vi "Interpolation Algo V1.vi"() -> (1 "SubRange":u16, 9 "MaxIndex":u16)   [LabVIEW 2013]
uses:
  Controls/Algorithm State.ctl
  <vilib>/Platform/TimedLoop/XDataNode/timing_clust.ctl
  <vilib>/Platform/TimedLoop/XDataNode/nitl_modes.ctl
  <vilib>/Platform/TimedLoop/XDataNode/wakeup.ctl
  <vilib>/rvi/Emulation/niFpgaSctlEmulationGetInTimedLoop.vi
  <vilib>/rvi/Emulation/niFpgaEmulationReportErrorSimple.vi
  <vilib>/rvi/Emulation/niFpgaGetClockAttributes.vi
  <vilib>/rvi/Emulation/niFpgaCriticalErrorInLSC.vi
  <vilib>/rvi/FIFO/Fifo_Resource/nirvififoEmulationReadFpgaImpl.vi
  <vilib>/rvi/DataTransferAndStorage/Container/Common/niFpgaContainerGetUniqueNameForEmu.vi
  <vilib>/rvi/interface/RandomDataEmulation/nirviRandomDataFPGAFIFO.vi
  <vilib>/rvi/interface/RandomDataEmulation/niFpgaRandomDataHandleErrors.vi
  <vilib>/rvi/Emulation/niFpgaProcessEmulError.vi
  LIDAR V2 Globals.vi
  <vilib>/rvi/FIFO/Fifo_Resource/nirvififoEmulationWriteFpgaImpl.vi
  <vilib>/rvi/Memory/Memory_Emulation/nirvimemoryFastEmulationFpgaImpl.vi
  <instcachedir>/0/nirvimemoryFastEmulationFpgaImpl_5FBAB50466BC4C939F684F8805638BFC.lvgen/nirvimemoryFastEmulationFpgaImpl_5FBAB50466BC4C939F684F8805638BFC_005.vi
  <vilib>/rvi/Memory/Memory_Emulation/nirvimemoryFastEmulation.vi
  <vilib>/rvi/Memory/Memory_Emulation/nirvimemoryEmulation.vi
  <instcachedir>/0/nirvimemoryFastEmulationFpgaImpl_5FBAB50466BC4C939F684F8805638BFC.lvgen/nirvimemoryFastEmulationFpgaImpl_5FBAB50466BC4C939F684F8805638BFC_007.vi
  <vilib>/Platform/TimedLoop/XDataNode/XDataNode.xnode
  <vilib>/rvi/DataTransferAndStorage/Container/XNode/niFpgaContainer.xnode
  <vilib>/rvi/FIFO/Fifo_Resource/nirvififoEmulationRead.vi
  <vilib>/rvi/interface/RandomDataEmulation/nirviRandomDataFpgaReadWriteTemplate.vi
  <vilib>/rvi/FIFO/Fifo_Resource/nirvififoEmulationWrite.vi
  <vilib>/rvi/FXPMathLib/FxpMul/XNode/nifxpmath_Multiplier.xnode
  <vilib>/rvi/FXPMathLib/FxpAdd/XNode/nifxpmath_Add.xnode
  <vilib>/Platform/TimedLoop/XDataNode/XDNodeRunTimeDep.lvlib
  <vilib>/rvi/FXPMathLib/sim/FxpSim.dll
panel:
  out "LedInfo":u16
  out "SumMaxValue":fxp<+/-,22,22>
  out "Buffer":fxp<+/-,22,22>[](array[numeric])
  out "AlgoState":T1
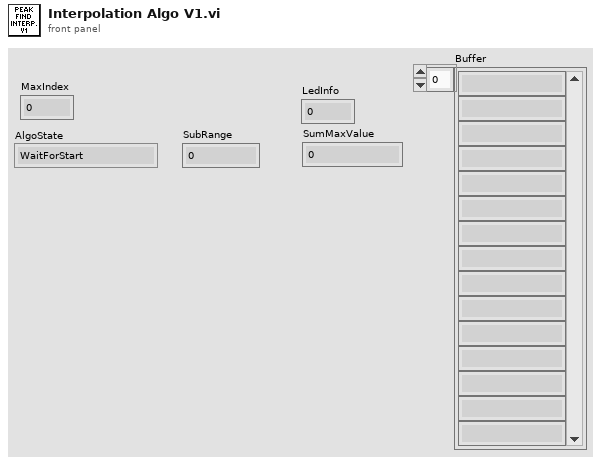
[diagram p1: front panel]
types:
  T1 = typedef "Algorithm State.ctl" = enum16{"WaitForStart", "GetNextSignalElement", "WaitForNextSignalElem", "MultWithSinc", "CalcMax"}
  T2 = typedef "XDNodeRunTimeDep.lvlib/timing_clust.ctl" = cluster{"Expected End [f-1]":u64, "Actual End [f-1]":u64, "Finished Late? [f-1]":bool, "Expected End [i-1]":u64, "Actual End [i-1]":u64, "Finished Late? [i-1]":bool, "Expected Start [i]":u64, "Actual Start [i]":u64, "Expected Start [f]":u64, "Actual Start [f]":u64, "Source Name":string, "Structure Name":string, "Period":i64, "Deadline":i64, "Offset":i64, "Start":i64, "Priority":i32, "Timeout":i32, "Mode":T3, "Wakeup Reason":T4, "Error":errorcluster, "Source Type":string, "Secondary Source Type":string, "Global End Time":u64, "Global Start Time":u64, "Frame Duration":u64, "Iteration Duration":u64, "Assigned CPU":i32, "I/O Scan Engine Mode":u32}
  T3 = typedef "XDNodeRunTimeDep.lvlib/nitl_modes.ctl" = enum32{"No Change", "Process missed periods, maintain original phase", "Discard missed periods, maintain original phase", "Process missed periods, ignore original phase", "Discard missed periods, ignore original phase"}
  T4 = typedef "XDNodeRunTimeDep.lvlib/wakeup.ctl" = enum32{"Normal", "Aborted", "Asynchronous wakeup", "Timing source error", "Timed loop error", "Timeout"}
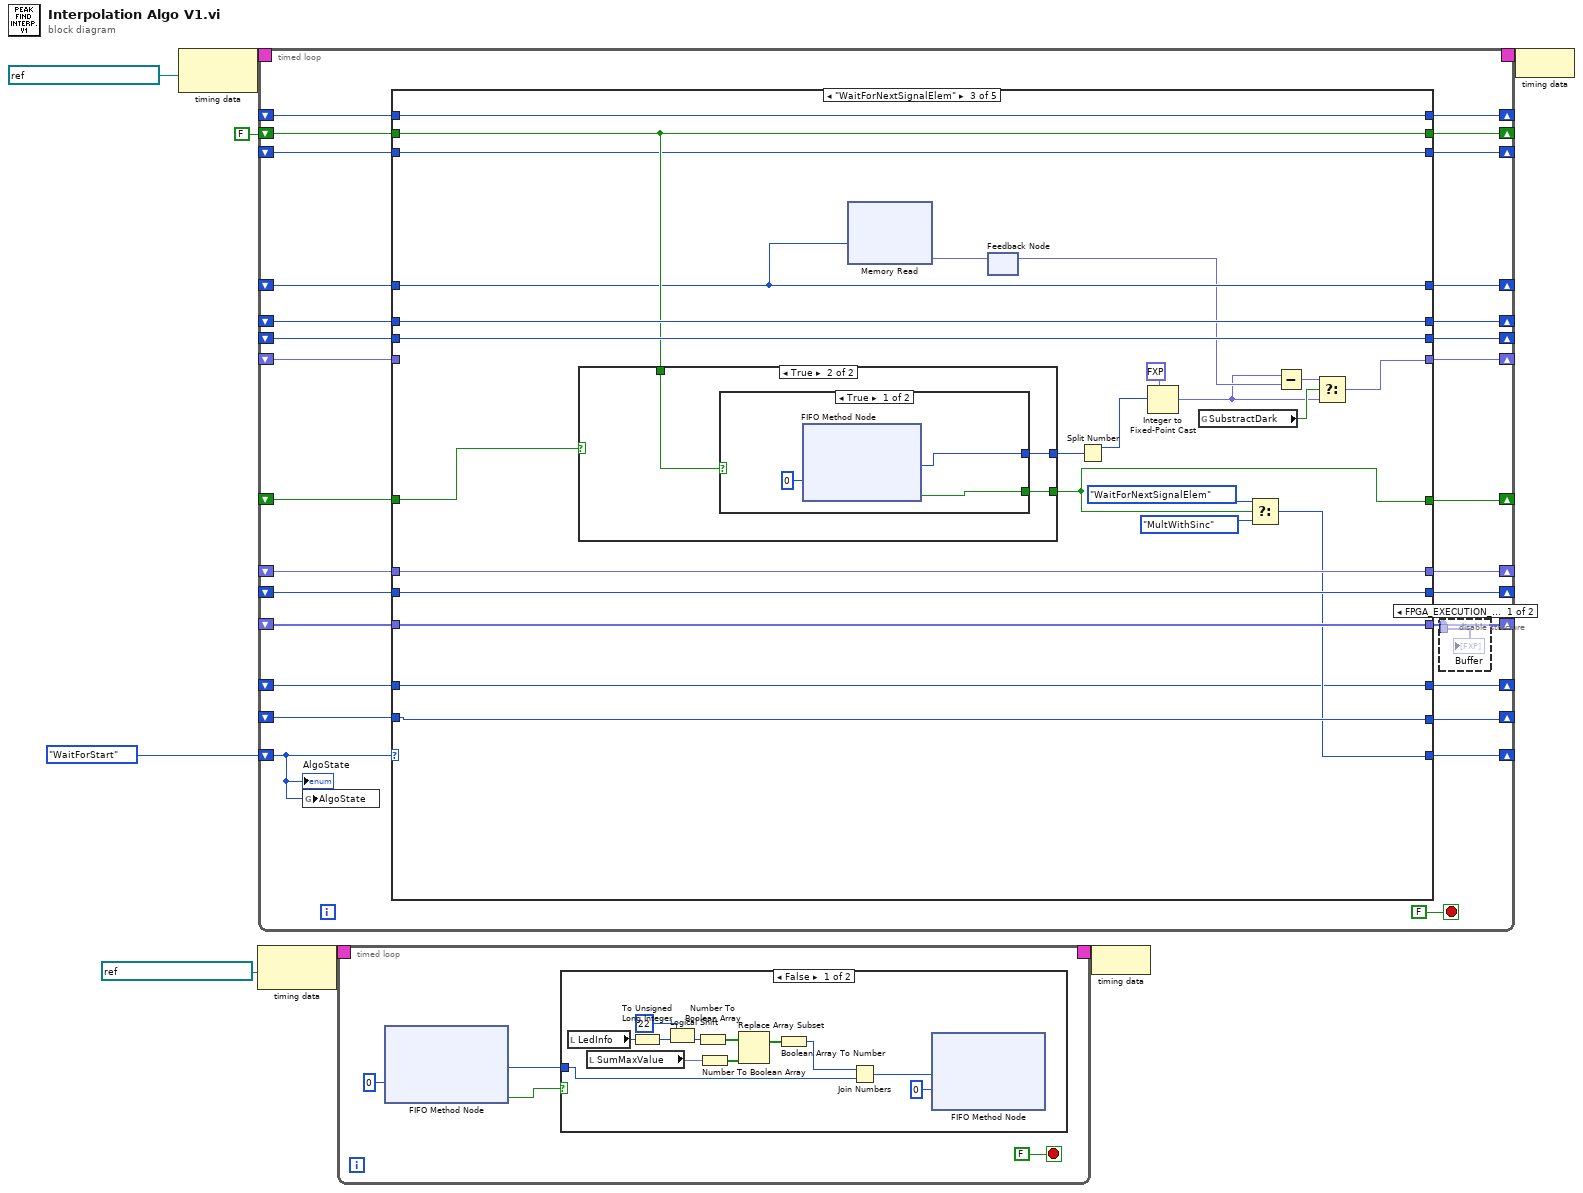
[diagram p0: block diagram]
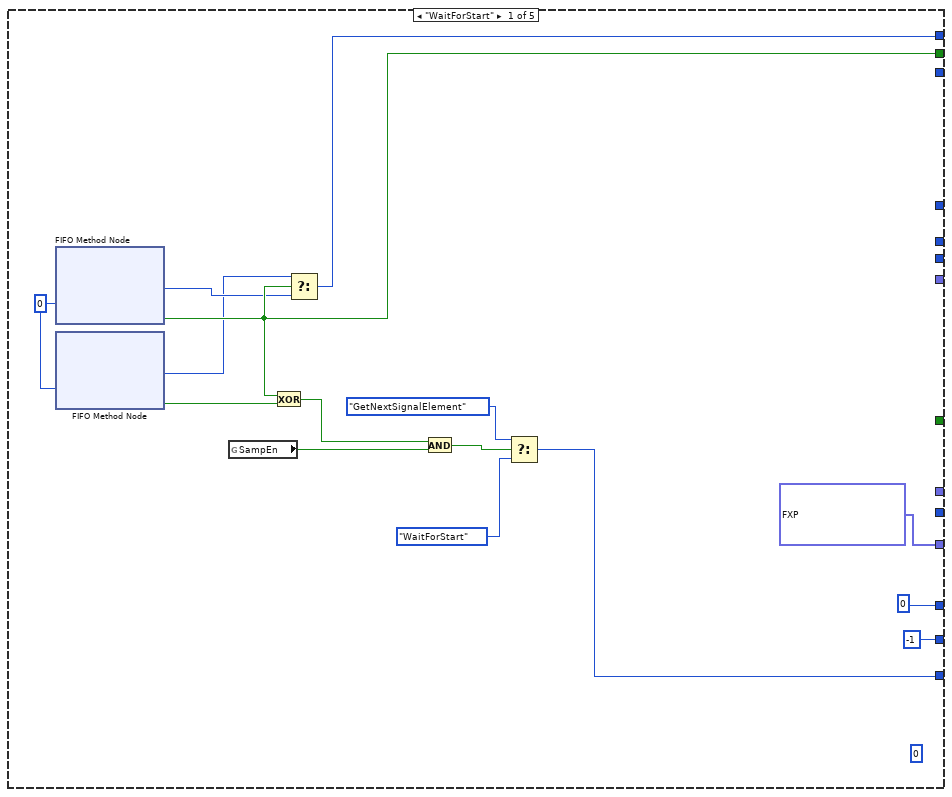
[diagram p4: hidden frame]
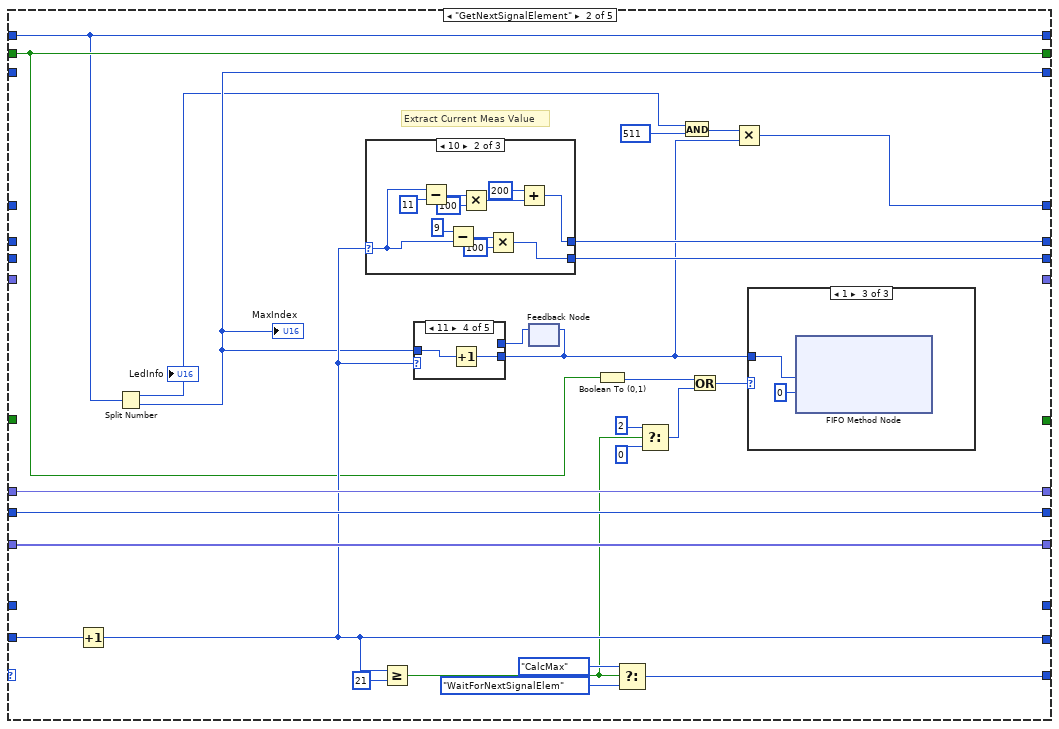
[diagram p5: hidden frame]
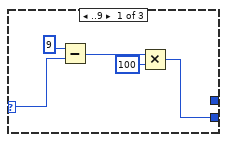
[diagram p6: hidden frame]
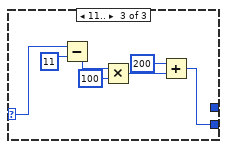
[diagram p7: hidden frame]
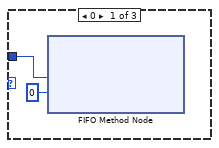
[diagram p8: hidden frame]
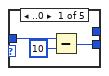
[diagram p10: hidden frame]
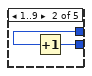
[diagram p11: hidden frame]
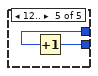
[diagram p13: hidden frame]
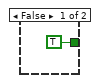
[diagram p14: hidden frame]
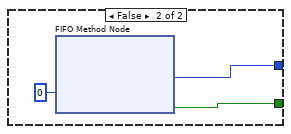
[diagram p15: hidden frame]
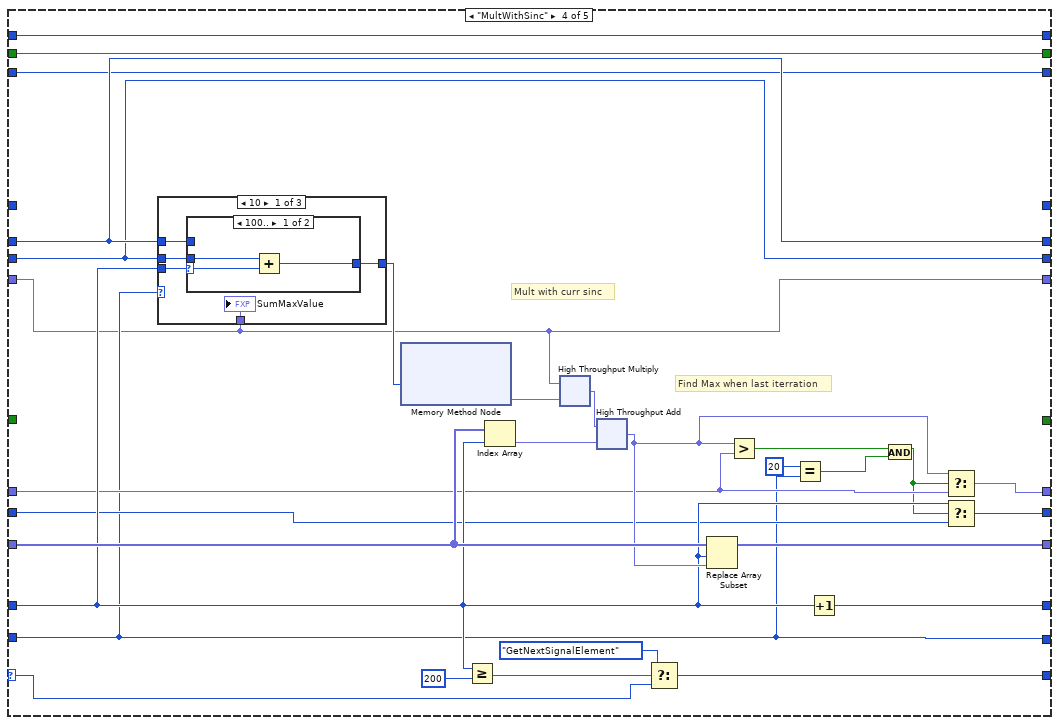
[diagram p16: hidden frame]
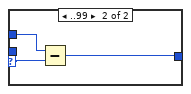
[diagram p17: hidden frame]
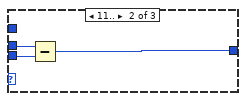
[diagram p18: hidden frame]
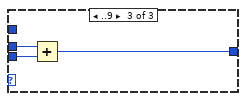
[diagram p19: hidden frame]
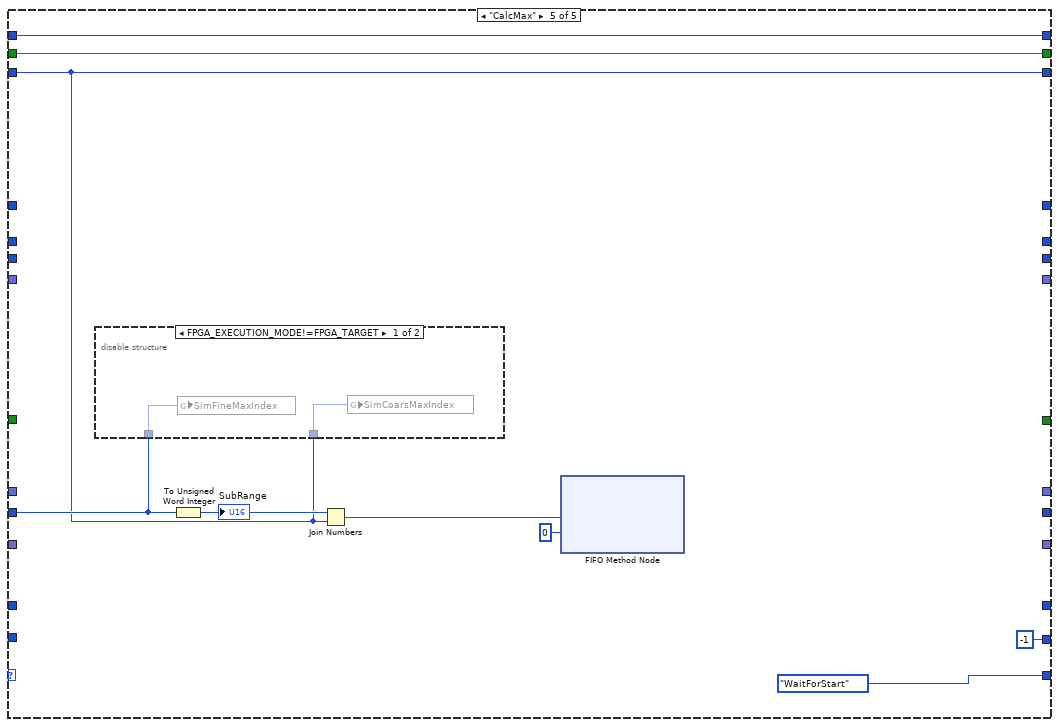
[diagram p20: hidden frame]
diagram:
  n1 = node-c288(refnum<k21> "40 MHz Onboard Clock" ("Source Name")) -> (w7:T2)
  n2 = node-c288(refnum<k21> "40 MHz Onboard Clock" ("Source Name")) -> (w4:T2)
  n3 = timed-loop {
    shift-right: [w33] -> _
    shift-left: Algorithm_State."WaitForStart" ("AlgoState") -> [w19]
    shift-right: [w36] -> _
    shift-left: _ -> [w37]
    shift-right: [w35] -> _
    shift-left: _ -> [w34]
    shift-right: [w32] -> _
    shift-left: _ -> [w30]
    shift-right: [w31] -> _
    shift-left: _ -> [w29]
    shift-right: [w28] -> _
    shift-left: _ -> [w27]
    shift-right: [w26] -> _
    shift-left: _ -> [w25]
    shift-right: [w24] -> _
    shift-left: _ -> [w21]
    shift-right: [w23] -> _
    shift-left: _ -> [w22]
    timing: w7 -> [_]
    timing-out: [_] -> w6
    shift-right: [w18] -> _
    shift-left: FALSE ("Timed Out?") -> [w17]
    shift-right: [w16] -> _
    shift-left: _ -> [w15]
    shift-right: [w14] -> _
    shift-left: _ -> [w13]
    shift-right: [w12] -> _
    shift-left: _ -> [w11]
    shift-right: [w10] -> _
    shift-left: _ -> [w9]
    stop <- FALSE stop-if-true
    n4 = global write "LIDAR V2 Globals.vi" "AlgoState"(w19) -> ()
    n5 = case shown="\"WaitForNextSignalElem\"" w19 {
      selector: w19 -> [_ _ _ w179 _]
      tunnel: w37 -> [_ w76 w137 w173 _]
      tunnel: [fxp<+/-,22,22>[] [0.0, 0.0, 0.0, 0.0, 0.0, 0.0, 0.0, 0.0, 0.0, 0.0, 0.0, 0.0, 0.0, 0.0, 0.0, 0.0, 0.0, 0.0, 0.0, 0.0, 0.0, 0.0, 0.0, 0.0, 0.0, 0.0, 0.0, 0.0, 0.0, 0.0, 0.0, 0.0, 0.0, 0.0, 0.0, 0.0, 0.0, 0.0, 0.0, 0.0, 0.0, 0.0, 0.0, 0.0, 0.0, 0.0, 0.0, 0.0, 0.0, 0.0, 0.0, 0.0, 0.0, 0.0, 0.0, 0.0, 0.0, 0.0, 0.0, 0.0, 0.0, 0.0, 0.0, 0.0, 0.0, 0.0, 0.0, 0.0, 0.0, 0.0, 0.0, 0.0, 0.0, 0.0, 0.0, 0.0, 0.0, 0.0, 0.0, 0.0, 0.0, 0.0, 0.0, 0.0, 0.0, 0.0, 0.0, 0.0, 0.0, 0.0, 0.0, 0.0, 0.0, 0.0, 0.0, 0.0, 0.0, 0.0, 0.0, 0.0, 0.0, 0.0, 0.0, 0.0, 0.0, 0.0, 0.0, 0.0, 0.0, 0.0, 0.0, 0.0, 0.0, 0.0, 0.0, 0.0, 0.0, 0.0, 0.0, 0.0, 0.0, 0.0, 0.0, 0.0, 0.0, 0.0, 0.0, 0.0, 0.0, 0.0, 0.0, 0.0, 0.0, 0.0, 0.0, 0.0, 0.0, 0.0, 0.0, 0.0, 0.0, 0.0, 0.0, 0.0, 0.0, 0.0, 0.0, 0.0, 0.0, 0.0, 0.0, 0.0, 0.0, 0.0, 0.0, 0.0, 0.0, 0.0, 0.0, 0.0, 0.0, 0.0, 0.0, 0.0, 0.0, 0.0, 0.0, 0.0, 0.0, 0.0, 0.0, 0.0, 0.0, 0.0, 0.0, 0.0, 0.0, 0.0, 0.0, 0.0, 0.0, 0.0, 0.0, 0.0, 0.0, 0.0, 0.0, 0.0, 0.0, 0.0, 0.0, 0.0, 0.0, 0.0, 0.0, 0.0, 0.0, 0.0, 0.0, 0.0, 0.0] ("Buffer") w76 w137 w176 _] -> w36
      tunnel: [i16 -1 w69 w136 w156 i16 -1] -> w35
      tunnel: w34 -> [_ w72 w136 w156 _]
      tunnel: [w48 w67 w133 w177 Algorithm_State."WaitForStart" ("AlgoState")] -> w33
      tunnel: [_ w74 w141 w172 _] -> w32
      tunnel: [_ w73 w140 w171 _] -> w31
      tunnel: w30 -> [_ _ w141 w172 _]
      tunnel: w29 -> [_ _ w140 w171 _]
      tunnel: [_ _ w117 w155 _] -> w28
      tunnel: w27 -> [_ _ _ w155 _]
      tunnel: [u16 0 _ w130 w158 _] -> w26
      tunnel: w25 -> [_ _ w130 w166 _]
      tunnel: [_ w70 w138 w169 _] -> w24
      tunnel: [_ w71 w139 w168 _] -> w23
      tunnel: w22 -> [_ w71 w139 w165 _]
      tunnel: w21 -> [_ w70 w138 w164 w204]
      tunnel: [w42 w61 w129 w154 w200] -> w18
      tunnel: w17 -> [_ w61 w129 w154 w200]
      tunnel: [_ w59 w128 w153 w199] -> w16
      tunnel: w15 -> [_ _ w128 w153 w199]
      tunnel: [w39 w60 w127 w152 w198] -> w14
      tunnel: w13 -> [_ w60 w127 w152 w198]
      tunnel: [_ w54 w124 _ _] -> w12
      tunnel: w11 -> [_ _ w124 _ _]
      tunnel: [_ _ w120 _ _] -> w10
      tunnel: w9 -> [_ _ w121 _ _]
      frame "WaitForStart" {
        w44 = 0 ("Timeout")
        (unwired) u8 0
        n6 = xnode ("FIFO Method Node")("Timeout"=w44) -> ("Element"=w41:u32, "Timed Out?"=w42:bool)  [unwired: 1 in, 1 out]
        n7 = xnode ("FIFO Method Node")("Timeout"=w44) -> ("Element"=w40:u32, "Timed Out?"=w43:bool)  [unwired: 1 in, 1 out]
        n8 = global read "LIDAR V2 Globals.vi" "SampEn"() -> (w46:bool)
        n9 = Exclusive Or(1:w43, 2:w42) -> (0:w45:bool)
        n10 = Select(t=w40, s=w42, f=w41) -> (s? t:f=w39:u32)
        n11 = And(x=w45, y=w46) -> (x .and. y?=w50:bool)
        n12 = Select(t=Algorithm_State."GetNextSignalElement" ("AlgoState"), s=w50, f=Algorithm_State."WaitForStart" ("AlgoState")) -> (s? t:f=w48:T1)
      }
      frame "GetNextSignalElement" {
        # "Extract Current Meas Value"
        n13 = Increment(x=w72) -> (x+1=w69:i16)
        n14 = Split Number(x=w60) -> (hi(x)=w58:u16, lo(x)=w59:u16)
        "MaxIndex" <- w59
        "LedInfo" <- w58
        n15 = case shown="10" w69 {
          selector: w69 -> [w80 w86 w96]
          tunnel: [w81 w92 w97] -> w73
          tunnel: [_ w85 _] -> w74
          frame ..9 {
            n16 = Subtract(x=9 ("y"), y=w80) -> (x-y=w83:i32)
            n17 = Multiply(x=w83, y=100) -> (x*y=w81:i32)
          }
          frame 10 {
            n18 = Subtract(x=w86, y=11) -> (x-y=w87:i32)
            n19 = Subtract(x=9 ("y"), y=w86) -> (x-y=w94:i32)
            n20 = Multiply(x=w87, y=100) -> (x*y=w90:i32)
            n21 = Multiply(x=w94, y=100) -> (x*y=w92:i32)
            n22 = Add(x=200, y=w90) -> (x+y=w85:i32)
          }
          frame 11.. {
            n23 = Subtract(x=w96, y=11) -> (x-y=w98:i32)
            n24 = Multiply(x=w98, y=100) -> (x*y=w101:i32)
            n25 = Add(x=200, y=w101) -> (x+y=w97:i32)
          }
        }
        n26 = Greater Or Equal?(x=w69, y=i16 21) -> (x >= y?=w66:bool)
        n27 = feedback #1() -> (w77:u16)  [unwired: 1 in]
        n28 = case shown="11" w69 {
          tunnel: [w107 w110 w112 w114 w115] -> w55
          tunnel: w77 -> [_ w111 _ _ w116]
          tunnel: w59 -> [w108 _ w112 w113 _]
          frame ..0 {
            n29 = Subtract(x=w108, y=u16 10) -> (x-y=w107:u16)
          }
          frame 1..9 {
            n30 = Increment(x=w111) -> (x+1=w110:u16)
          }
          frame 10 {
          }
          frame 11 {
            n31 = Increment(x=w113) -> (x+1=w114:u16)
          }
          frame 12.. {
            n32 = Increment(x=w116) -> (x+1=w115:u16)
          }
        }
        n33 = feedback-in #1(w55) -> ()
        n34 = Boolean To (0,1)(Boolean=w61) -> (0, 1=w68:i16)
        n35 = Select(t=Algorithm_State."CalcMax", s=w66, f=Algorithm_State."WaitForNextSignalElem" ("AlgoState")) -> (s? t:f=w67:T1)
        n36 = Select(t=i16 2, s=w66, f=i16 0) -> (s? t:f=w63:i16)
        n37 = And(x=w58, y=u16 511) -> (x .and. y?=w56:u16)
        n38 = Or(x=w68, y=w63) -> (x .or. y?=w62:i16)
        n39 = Multiply(x=w56, y=w55) -> (x*y=w54:u16)
        n40 = case shown="1" w62 {
          tunnel: w55 -> [w103 _ w105]
          frame 0 {
            n41 = xnode ("FIFO Method Node")("Element"=w103, "Timeout"=0) -> ()  [unwired: 1 in, 2 out]
          }
          frame Default {
          }
          frame 1 {
            n42 = xnode ("FIFO Method Node")("Element"=w105, "Timeout"=0) -> ()  [unwired: 1 in, 2 out]
          }
        }
      }
      frame "WaitForNextSignalElem" {
        n43 = case shown="True" w121 {
          tunnel: [_ w145] -> w132
          tunnel: w129 -> [_ w144]
          tunnel: [TRUE ("Timed Out?") w143] -> w120
          frame False {
          }
          frame True {
            n44 = case shown="True" w144 {
              tunnel: [w147 w150] -> w143
              tunnel: [w146 w149] -> w145
              frame True {
                n45 = xnode ("FIFO Method Node")("Timeout"=0) -> ("Element"=w146:u64, "Timed Out?"=w147:bool)  [unwired: 1 in, 1 out]
              }
              frame False {
                n46 = xnode ("FIFO Method Node")("Timeout"=0) -> ("Element"=w149:u64, "Timed Out?"=w150:bool)  [unwired: 1 in, 1 out]
              }
            }
          }
        }
        n47 = xnode ("Memory Read")("Address"=w124) -> ("Data"=w123:fxp<+/-,22,22>)  [unwired: 1 in, 1 out]
        n48 = feedback-in #2(w123) -> ()
        n49 = feedback #2() -> (w122:fxp<+/-,22,22>)  [unwired: 1 in]
        n50 = Split Number(x=w132) -> (hi(x)=w119:u32)  [unwired: 1 out]
        n51 = Integer to Fixed-Point Cast(fixed-point type=fxp<+/-,22,22> 0.0, integer=w119) -> (fixed-point=w118:fxp<+/-,22,22>)
        n52 = global read "LIDAR V2 Globals.vi" "SubstractDark"() -> (w125:bool)
        n53 = Select(t=Algorithm_State."WaitForNextSignalElem" ("AlgoState"), s=w120, f=Algorithm_State."MultWithSinc" ("AlgoState")) -> (s? t:f=w133:T1)
        n54 = Subtract(x=w118, y=w122) -> (x-y=w126:fxp<+/-,23,23>)
        n55 = Select(t=w126, s=w125, f=w118) -> (s? t:f=w117:fxp<+/-,23,23>)
      }
      frame "MultWithSinc" {
        # "Find Max when last iterration"
        # "Mult with curr sinc"
        n56 = case shown="10" w156 {
          tunnel: w166 -> [w183 w194 w197]
          tunnel: w171 -> [w185 w193 w196]
          tunnel: [w184 w192 w195] -> w160
          tunnel: w172 -> [w182 _ _]
          tunnel: w155 -> [w181 _ _]
          frame 10 {
            n57 = case shown="100.." w183 {
              selector: w183 -> [w186 w191]
              tunnel: w185 -> [w188 _]
              tunnel: [w187 w190] -> w184
              tunnel: w182 -> [_ w189]
              frame 100.. {
                n58 = Add(x=w188, y=w186) -> (x+y=w187:i32)
              }
              frame ..99 {
                n59 = Subtract(x=w189, y=w191) -> (x-y=w190:i32)
              }
            }
            "SumMaxValue" <- w181
          }
          frame 11.. {
            n60 = Subtract(x=w193, y=w194) -> (x-y=w192:i32)
          }
          frame ..9 {
            n61 = Add(x=w196, y=w197) -> (x+y=w195:i32)
          }
        }
        n62 = xnode ("Memory Method Node")("Address"=w160) -> ("Data"=w159:fxp<+/-,22,1>)  [unwired: 1 in, 1 out]
        n63 = Greater Or Equal?(x=w166, y=u16 200) -> (x >= y?=w157:bool)
        n64 = Index Array(array=w173, index=w166) -> (element=w174:fxp<+/-,22,22>)
        n65 = xnode ("High Throughput Multiply")("x"=w155, "y"=w159) -> ("x*y"=w175:fxp<+/-,22,22>)
        n66 = xnode ("High Throughput Add")("x"=w175, "y"=w174) -> ("x+y"=w167:fxp<+/-,22,22>)
        n67 = Select(t=Algorithm_State."GetNextSignalElement", s=w157, f=w179) -> (s? t:f=w177:T1)
        n68 = Replace Array Subset(array=w173, new element=w167, index=w166) -> (w176:fxp<+/-,22,22>[])
        n69 = Greater?(x=w167, y=w165) -> (0:w170:bool)
        n70 = Equal?(x=i16 20, y=w156) -> (x = y?=w161:bool)
        n71 = Increment(x=w166) -> (x+1=w158:u16)
        n72 = And(x=w170, y=w161) -> (x .and. y?=w163:bool)
        n73 = Select(t=w167, s=w163, f=w165) -> (s? t:f=w168:fxp<+/-,22,22>)
        n74 = Select(t=w166, s=w163, f=w164) -> (s? t:f=w169:u16)
      }
      frame "CalcMax" {
        n75 = disable-structure shown="FPGA_EXECUTION_MODE!=FPGA_TARGET" {
          disable-tunnel: w199 -> [w208 _]
          disable-tunnel: w204 -> [w207 _]
          frame condition #0 {
            n76 = global write "LIDAR V2 Globals.vi" "SimFineMaxIndex"(w207) -> ()
            n77 = global write "LIDAR V2 Globals.vi" "SimCoarsMaxIndex"(w208) -> ()
          }
          frame condition #1 (active) {
          }
        }
        n78 = To Unsigned Word Integer(number=w204) -> (unsigned 16bit integer=w205:u16)
        "SubRange" <- w205
        n79 = Join Numbers(hi=w205, lo=w199) -> ((hi.lo)=w203:u32)
        n80 = xnode ("FIFO Method Node")("Element"=w203, "Timeout"=0) -> ()  [unwired: 1 in, 2 out]
      }
    }
    n81 = disable-structure shown="FPGA_EXECUTION_MODE!=FPGA_TARGET" {
      disable-tunnel: w36 -> [w38 _]
      frame condition #0 {
        "Buffer" <- w38
      }
      frame condition #1 (active) {
      }
    }
    "AlgoState" <- w19
  }
  n82 = timed-loop {
    timing: w4 -> [_]
    timing-out: [_] -> w3
    stop <- FALSE stop-if-true
    n83 = xnode ("FIFO Method Node")("Timeout"=0) -> ("Element"=w214:u32, "Timed Out?"=w211:bool)  [unwired: 1 in, 1 out]
    n84 = case shown="False" w211 {
      tunnel: w214 -> [w226 _]
      frame False {
        n85 = local read "LedInfo"() -> (w218:u16)
        n86 = local read "SumMaxValue"() -> (w220:fxp<+/-,22,22>)
        n87 = To Unsigned Long Integer(number=w218) -> (unsigned 32bit integer=w217:u32)
        n88 = Logical Shift(y=i16 22, x=w217) -> (x << y=w216:u32)
        n89 = Number To Boolean Array(number=w216) -> (Boolean array=w221:bool[])
        n90 = Number To Boolean Array(number=w220) -> (Boolean array=w222:bool[])
        n91 = Replace Array Subset(array=w221, new element=w222) -> (w223:bool[])  [unwired: 1 in]
        n92 = Boolean Array To Number(Boolean array=w223) -> (number=w219:u32)
        n93 = Join Numbers(hi=w219, lo=w226) -> ((hi.lo)=w225:u64)
        n94 = xnode ("FIFO Method Node")("Element"=w225, "Timeout"=0) -> ()  [unwired: 1 in, 2 out]
      }
      frame True {
      }
    }
  }
  n95 = node-c288(w3) -> ()
  n96 = node-c288(w6) -> ()
